vi "start.vi"(8 "error in (no error)":errorcluster, 11 "DL090211DAQScaffold in":refnum<class "DAQ_DL091205Readers.lvclass">) -> (0 "error out":errorcluster, 3 "DL090211DAQScaffold out":refnum<class "DAQ_DL091205Readers.lvclass">)   [LabVIEW 2010, in "DAQ_DL091205Readers.lvclass"]
uses:
  DAQ_DL091205Readers.lvclass
  DAQ_DL090211Scaffold/DAQ_DL090211Scaffold/DAQ_DL090211Scaffold.lvclass
  DAQ_DL091205Readers.lvclass/DAQ_DL091205Readers.ctl
  SignalReader/GenericSignalReader/GenericSignalReader/GenericSignalReader.lvclass
  common/classes/ErrorController/ErrorController/class_data.vi
  common/classes/ErrorController/ErrorController/ErrorController.lvclass
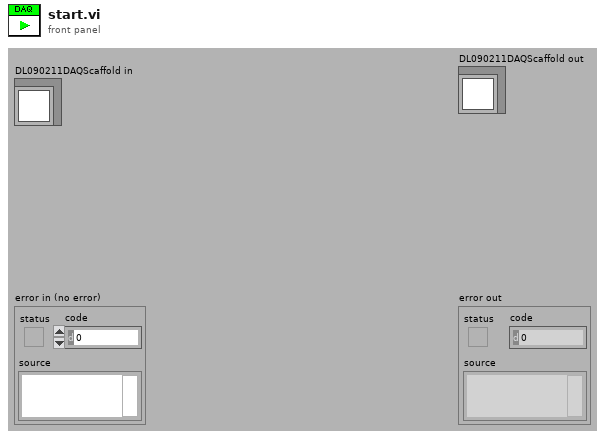
[diagram p1: front panel]
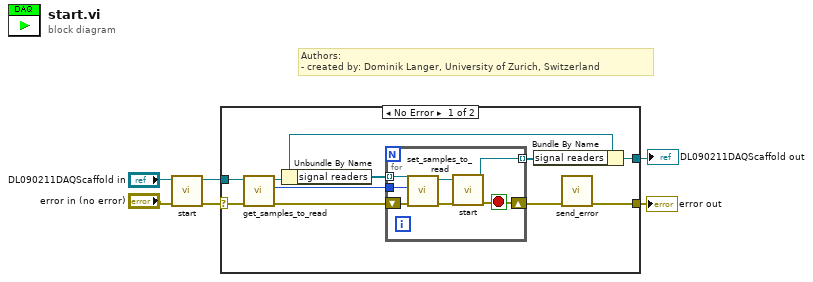
[diagram p0: block diagram]
diagram:
  # "Authors: \n- created by: Dominik Langer, University of Zurich, Switzerland"
  n1 = call-parent "start.vi"("error in (no error)"="error in (no error)", "DL090211DAQScaffold in"="DL090211DAQScaffold in") -> ("error out"=w4:errorcluster, "DL090211DAQScaffold out"=w3:refnum<class "DAQ_DL091205Readers.lvclass">)  [unwired: 8 in]
  n2 = case shown="No Error" w4 {
    selector: w4 -> [w13 w25]
    tunnel: w3 -> [w11 w24]
    tunnel: [w8 w25] -> w2
    tunnel: [w14 w24] -> w1
    frame No Error {
      n3 = call-dynamic "get_samples_to_read.vi"("error in (no error)"=w13, "GenericDAQ.lvclass in"=w11) -> ("error out"=w12:errorcluster, "samples to read"=w9:i64, "GenericDAQ.lvclass out"=w10:refnum<class "DAQ_DL091205Readers.lvclass">)  [unwired: 7 in]
      n4 = Unbundle By Name(w10) -> ("signal readers"=w16:refnum<class "GenericSignalReader.lvclass">[])
      n5 = for {
        tunnel: w16 -> [w19] mode=indexing
        tunnel: [w23] -> w15 mode=indexing
        tunnel: w9 -> [w20]
        shift-right: [w17] -> w7
        shift-left: w12 -> [w22]
        stop <- w17 stop-if-true
        n6 = call-dynamic "set_samples_to_read.vi"("error in (no error)"=w22, "samples to read"=w20, "GenericSignalReader in"=w19) -> ("error out"=w21:errorcluster, "GenericSignalReader out"=w18:refnum<class "GenericSignalReader.lvclass">)  [unwired: 7 in]
        n7 = call-dynamic "start.vi"("error in (no error)"=w21, "GenericSignalReader in"=w18) -> ("error out"=w17:errorcluster, "GenericSignalReader out"=w23:refnum<class "GenericSignalReader.lvclass">)  [unwired: 8 in]
      }
      n8 = Bundle By Name(cluster=w10, "signal readers"=w15) -> (w14:refnum<class "DAQ_DL091205Readers.lvclass">)
      n9 = call "send_error.vi"("error in (no error)"=w7) -> ("error out"=w8:errorcluster)  [unwired: 10 in]
    }
    frame Error {
    }
  }
  "error out" <- w2
  "DL090211DAQScaffold out" <- w1
